vi "nPr_nCr.vi"() -> ()   [LabVIEW 2024]
panel:
  out "Numeric":dbl
  out "Numeric 2":dbl
  in  "n 4":i32
  in  "n 3":i32
  in  "n 2":i32
  in  "n":i32
  # "nPr"
  # "nCr"
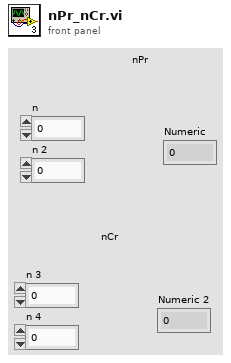
[diagram p1: front panel]
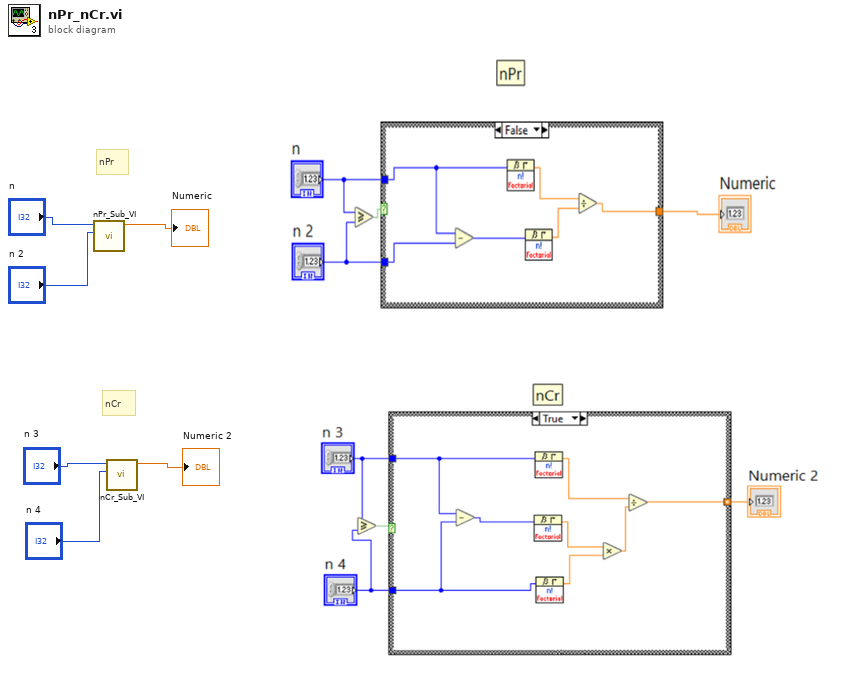
[diagram p0: block diagram]
diagram:
  # "nCr"
  # "nPr"
  n1 = call "nPr_Sub_VI.vi"("n 2"="n 2", "n"="n") -> ("Numeric"=→"Numeric":dbl)  [unwired: 9 in]
  n2 = call "nCr_Sub_VI.vi"("n 4"="n 4", "n 3"="n 3") -> ("Numeric 2"=→"Numeric 2":dbl)  [unwired: 9 in]
